vi "Start Server.vi"(8 "error in (no error)":errorcluster, 11 "GodotServer in":refnum<class "GodotServer.lvclass">) -> (0 "error out":errorcluster, 3 "GodotServer out":refnum<class "GodotServer.lvclass">)   [LabVIEW 2020, in "GodotLV.lvlib" / "GodotServer.lvclass"]
uses:
  GodotServer.lvclass
  GodotServer.lvclass/GodotServer.ctl
  <vilib>/IlluminatedG/IG HTTP Server/HTTP Server/Server/Server.lvclass
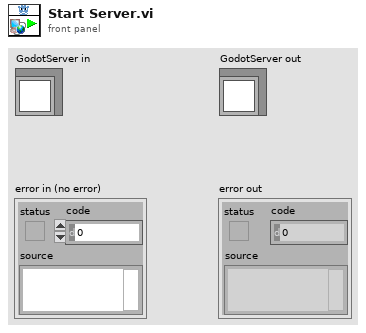
[diagram p1: front panel]
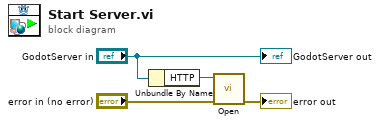
[diagram p0: block diagram]
diagram:
  n1 = Unbundle By Name("GodotServer in") -> ("HTTP"=w3:refnum<class "Server.lvclass">)
  n2 = call <vilib>:"Open.vi"("error in (no error)"="error in (no error)", "Server in"=w3) -> ("error out"=→"error out":errorcluster)  [unwired: 8 in, 1 out]
  "GodotServer out" <- "GodotServer in"
